vi "Testing Database UI.vi"() -> ()   [LabVIEW 2012, in "Architecture.lvlib" / "Database.lvclass"]
uses:
  Database.lvclass
  Database Record.ctl
  Database Action.ctl
panel:
  out "Timing Array":i16[](array[numeric])
  out "Database Records":T1[](array[typedef])
  out "error out":errorcluster
  in  "Database Action":T2
  in  "Database Record":T1
  in  "Database Records In":T1[](array[typedef])
  in  "error in (no error)":errorcluster
  in  "Stop Button":bool
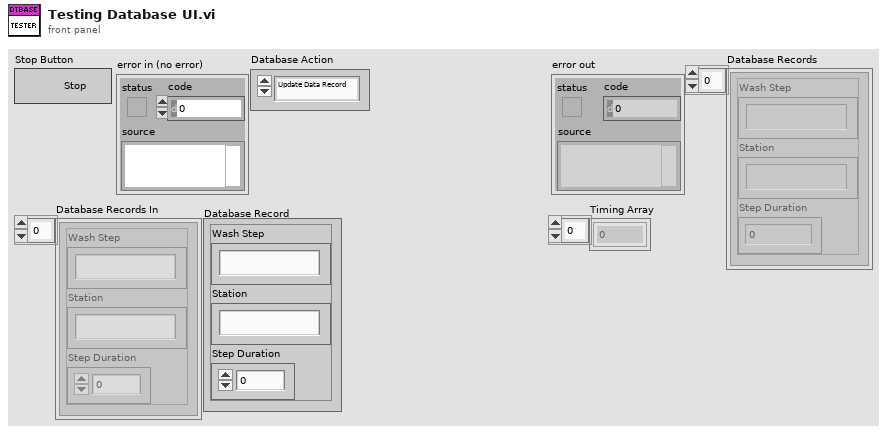
[diagram p1: front panel]
types:
  T1 = typedef "Architecture.lvlib/Database.lvclass/Database Record.ctl" = cluster{"Wash Step":string, "Station":string, "Step Duration":i16}
  T2 = typedef "Architecture.lvlib/Database.lvclass/Database Action.ctl" = enum16{"Update Data Record", "Insert New Data Record", "Query Timing Data", "Read Records", "Initialize"}
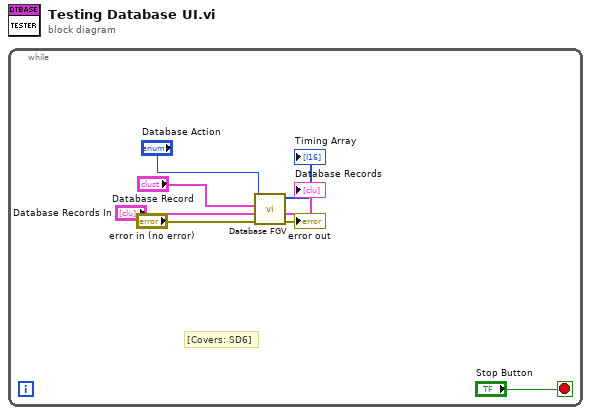
[diagram p0: block diagram]
diagram:
  n1 = while {
    stop <- "Stop Button" stop-if-true
    # "[Covers: SD6]"
    n2 = call "Database FGV.vi"("error in (no error)"="error in (no error)", "Database Records In"="Database Records In", "Database Record"="Database Record", "Database Action"="Database Action") -> ("error out"=→"error out":errorcluster, "Database Records"=→"Database Records":T1[], "Timing Array"=→"Timing Array":i16[])  [unwired: 5 in]
  }
